vi "timing harness--xml load.vi"() -> ()   [LabVIEW 2021]
uses:
  Material Theme/Material Theme.lvclass
panel:
  out "avg per loop (ms)":dbl
  in  "loops":i32=100
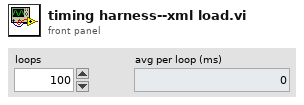
[diagram p1: front panel]
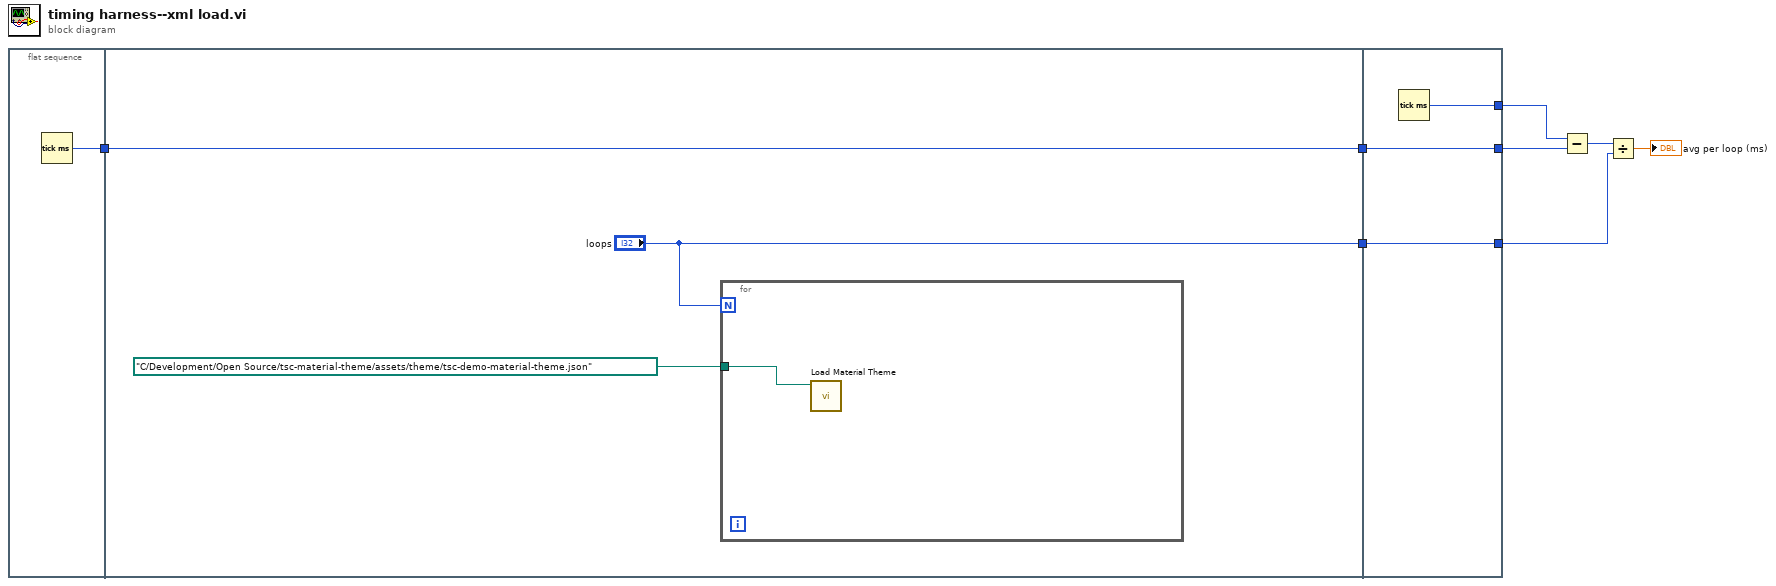
[diagram p0: block diagram]
diagram:
  n1 = flat-sequence {
    tunnel: [w9] -> w8
    tunnel: w8 -> [w11]
    tunnel: [w11] -> w7
    tunnel: ["loops"] -> w3
    tunnel: w7 -> [w16]
    tunnel: [w16] -> w6
    tunnel: [w15] -> w5
    tunnel: w3 -> [w14]
    tunnel: [w14] -> w2
    frame #0 {
      n2 = Tick Count (ms)() -> (millisecond timer value=w9:u32)
    }
    frame #1 {
      n3 = for {
        N: "loops" -> [_]
        tunnel: path "C:/Development/Open Source/tsc-material-theme/assets/theme/tsc-demo-material-theme.json" ("file path (use dialog)") -> [w13]
        n4 = call "Load Material Theme.vi"("file path"=w13) -> ()  [unwired: 9 in, 2 out]
      }
    }
    frame #2 {
      n5 = Tick Count (ms)() -> (millisecond timer value=w15:u32)
    }
  }
  n6 = Subtract(x=w5, y=w6) -> (x-y=w4:u32)
  n7 = Divide(x=w4, y=w2) -> (x/y=→"avg per loop (ms)":dbl)
